vi "FG Count.vi"(2 "FG Action (Read)":T1, 3 "Count in":i32) -> (1 "Count out":i32)   [LabVIEW 2009]
uses:
  FG Action (Read).ctl
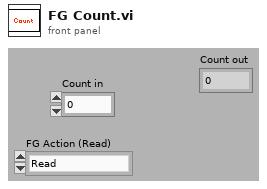
[diagram p1: front panel]
types:
  T1 = typedef "FG Action (Read).ctl" = enum16{"Read", "Write"}
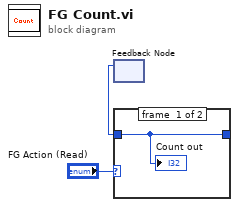
[diagram p0: block diagram]
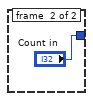
[diagram p2: hidden frame]
diagram:
  n1 = feedback #1() -> (w2:i32)  [unwired: 1 in]
  n2 = case shown="\"Write\"" "FG Action (Read)" {
    tunnel: [w4 "Count in"] -> w3
    tunnel: w2 -> [w4 _]
    frame #0 {
      "Count out" <- w4
    }
    frame #1 {
    }
  }
